vi "Read Image on Button.vi"(9 "image item":i32, 11 "File with Button":path) -> (0 "error out":errorcluster, 3 "png file out":path)   [LabVIEW 2018]
doc: "This example VI was obtained from this post. This strips out the saving profile and just reads the image on an existing button.\n\nhttps://forums.ni.com/t5/LabVIEW-APIs-Discussions/Set-TRUE-FALSE-Image-of-a-boolean-control-automatically-using/m-p/3419083/highlight/true#M868\n\n<b>WARNING</b>\nThis VI uses a dll call to the resource file for a LabVIEW VI/CTL - it is searching the binary data for the PNG images that the VI or CTL contains\n\n<b>Code Developed By:</b>\nTechnology Service Corporation\n1983 S Liberty Drive\nBloomington, IN 47403\nPhone: 812 558-7100\nwww.tsc.com/atcs\n\nDeveloper:\nDaniel Coons"
panel:
  out "Resources":string[](array[string])
  # "MNGI resources are 6 images\non buttons (pressed, hover, etc)\n\n-When set to a \"decal\", it should\nbe the only one"
  # "For DEBUG"
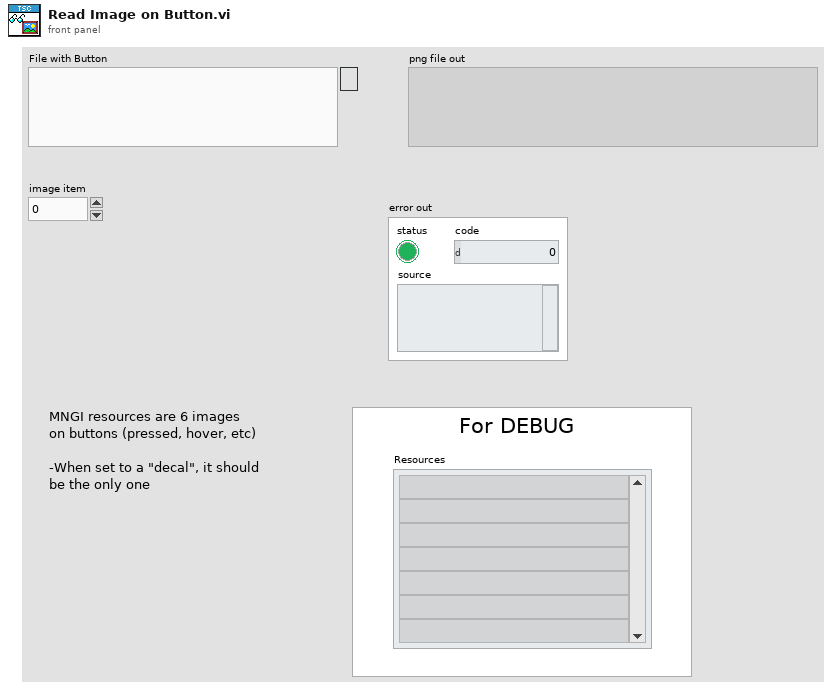
[diagram p1: front panel]
types:
  T1 = enum16{"open", "replace", "create", "open or create", "replace or create", "replace or create with confirmation"}
  T2 = cluster{"type":u32, "id":i32, "name":string, "binary data":string}[]
  T3 = cluster{"type":u32, "id":i32, "name":string, "binary data":string}
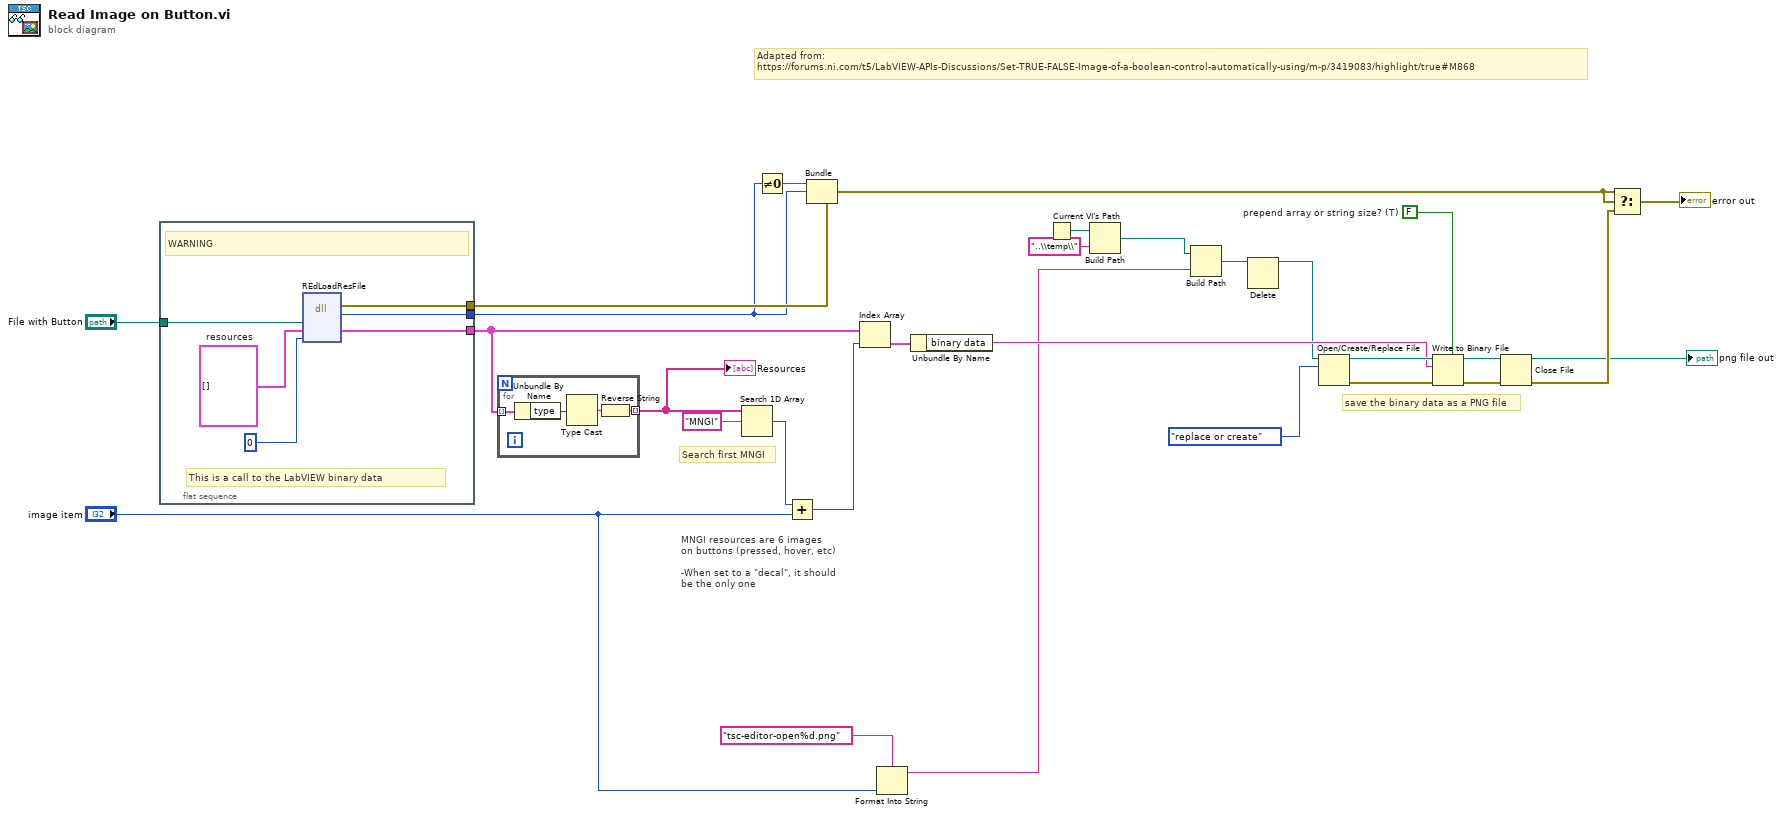
[diagram p0: block diagram]
diagram:
  w9 = FALSE  # prepend array or string size? (T)
  # "MNGI resources are 6 images\non buttons (pressed, hover, etc)\n\n-When set to a \"decal\", it should\nbe the only one"
  # "save the binary data as a PNG file"
  # "Adapted from:\nhttps://forums.ni.com/t5/LabVIEW-APIs-Discussions/Set-TRUE-FALSE-Image-of-a-boolean-control-automatically-using/m-p/3419083/highlight/true#M868"
  # "Search first MNGI"
  n1 = flat-sequence {
    tunnel: [w33] -> w29
    tunnel: [w32] -> w27
    tunnel: "File with Button" -> [w31]
    tunnel: [w30] -> w23
    frame #0 {
      w35 = T2 []  # resources
      # "This is a call to the LabVIEW binary data"
      # "WARNING"
      n2 = dll-call lib="LabVIEW" fn="REdLoadResFile"("path"=w31, "resources"=w35, "type"=0) -> (error out=w33:errorcluster, "return type"=w32:i32, "resources"=w30:T2)  [unwired: 3 in, 3 out]
    }
  }
  n3 = for {
    tunnel: w23 -> [w39] mode=indexing
    tunnel: [w36] -> w7 mode=indexing
    n4 = Unbundle By Name(w39) -> ("type"=w37:u32)
    n5 = Type Cast(x=w37) -> (*(type *) &x=w38:string)  [unwired: 1 out]
    n6 = Reverse String(1:w38) -> (0:w36:string)
  }
  "Resources" <- w7
  n7 = Search 1D Array(1D array=w7, element="MNGI") -> (index of element=w21:i32)  [unwired: 1 out]
  n8 = Not Equal To 0?(x=w27) -> (x != 0?=w28:bool)
  n9 = Add(x=w21, y="image item") -> (x+y=w22:i32)
  n10 = Bundle(cluster=w29, "status"=w28, "code"=w27) -> (w25:errorcluster)  [unwired: 1 out]
  n11 = Index Array(array=w23, index=w22) -> (element=w20:T3)
  n12 = Format Into String(format string="tsc-editor-open%d.png", "image item") -> (resulting string=w6:string)  [unwired: 2 in, 1 out]
  n13 = Unbundle By Name(w20) -> ("binary data"=w15:string)
  n14 = Current VI's Path() -> (path=w4:path)
  n15 = Build Path(base path=w4, name or relative path="..\\temp\\") -> (appended path=w2:path)
  n16 = Build Path(base path=w2, name or relative path=w6) -> (appended path=w19:path)
  n17 = Delete(path (use dialog)=w19) -> (deleted path=w10:path)  [unwired: 4 in, 2 out]
  n18 = Open/Create/Replace File(file path (use dialog)=w10, operation (0:open)=T1."replace or create") -> (refnum out=w16:refnum<file>, error out=w17:errorcluster)  [unwired: 4 in, 1 out]
  n19 = Write to Binary File(file (use dialog)=w16, data=w15, error in=w17, 5:w9) -> (refnum out=w13:refnum<file>, error out=w14:errorcluster)  [unwired: 2 in, 1 out]
  n20 = Close File(refnum=w13, error in=w14) -> (path=→"png file out":path, error out=w12:errorcluster)
  n21 = Select(t=w25, s=w25, f=w12) -> (s? t:f=→"error out":errorcluster)
